vi "QD_Error_Logger.vi"(0 "State_and_Data_In":T1, 1 "Max_Queue_Size_In":i32=-1, 2 "Queue_Name_In":string, 5 "State_and_Data_N_In":T1[](array[typedef]), 7 "Time_Out_In_ms (-1)":i32, 11 "Error_In":errorcluster, 13 "Queue_Operation":T2=enum."Flush") -> (4 "State_and_Data_Out":T1, 15 "Error_Out":errorcluster)   [LabVIEW 2021]
doc: "Used to transfer data from one vi to another using queue."
uses:
  Controls/Queue_Operation_Select.ctl
  Controls/State_and_Data.ctl
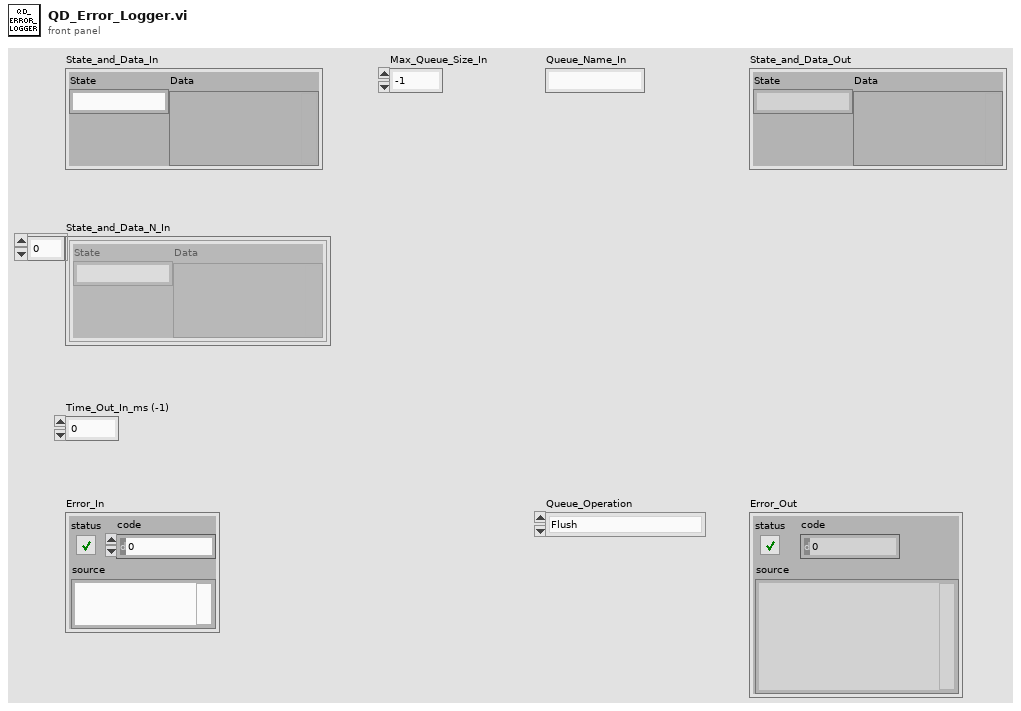
[diagram p1: front panel]
types:
  T1 = typedef "State_and_Data.ctl" = cluster{"State":string, "Data":variant}
  T2 = typedef "Queue_Operation_Select.ctl" = enum16{"Obtain_Queue", "Enqueue", "Enqueue_First", "Enqueue_N", "Lossy_Enqueue", "Preview", "Queue_Status", "Dequeue", "Flush", "Release_Queue"}
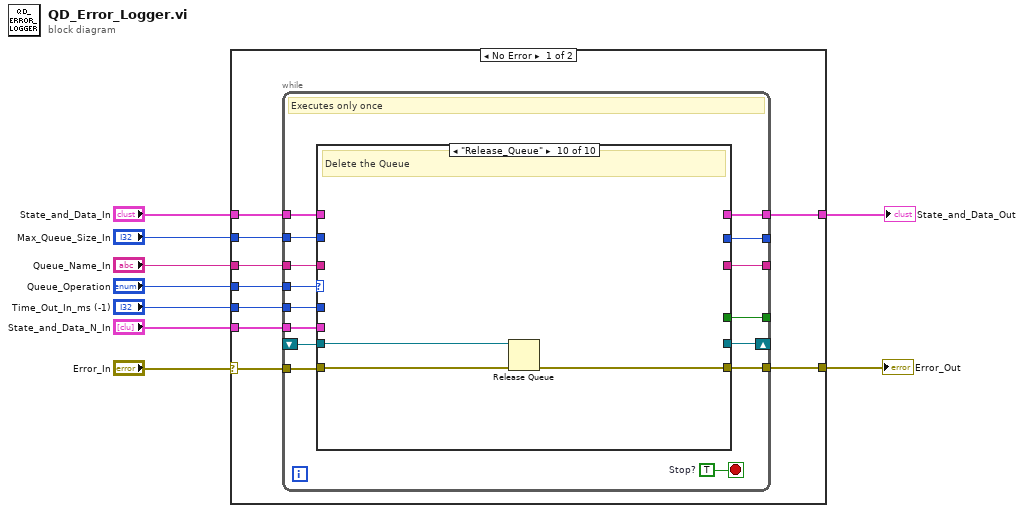
[diagram p0: block diagram]
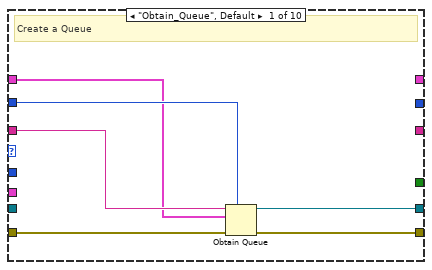
[diagram p2: hidden frame]
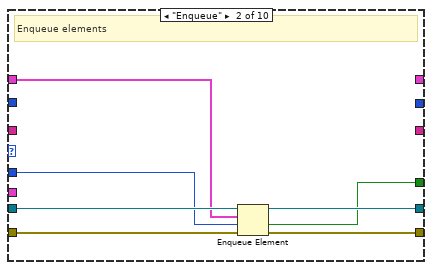
[diagram p3: hidden frame]
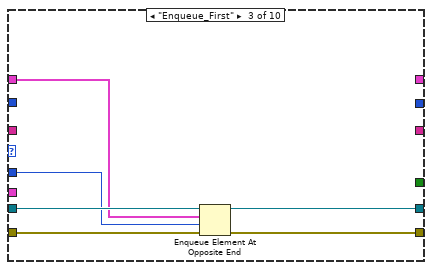
[diagram p4: hidden frame]
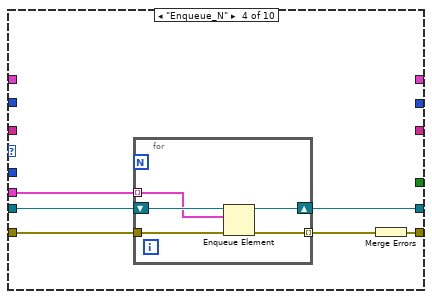
[diagram p5: hidden frame]
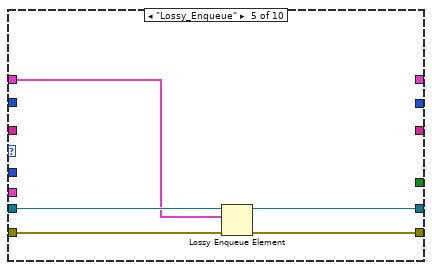
[diagram p6: hidden frame]
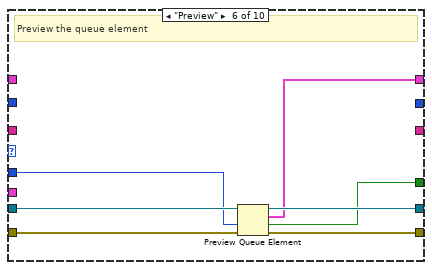
[diagram p7: hidden frame]
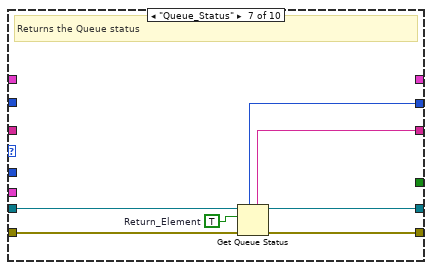
[diagram p8: hidden frame]
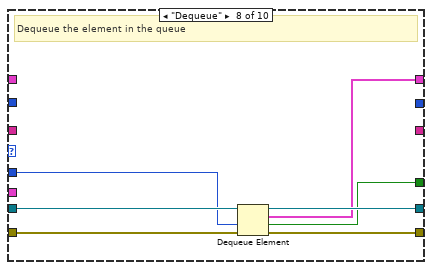
[diagram p9: hidden frame]
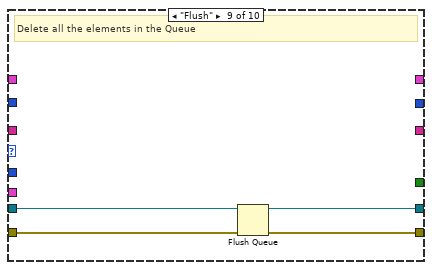
[diagram p10: hidden frame]
diagram:
  n1 = case shown="No Error" "Error_In" {
    selector: "Error_In" -> [w10 w97]
    tunnel: "Max_Queue_Size_In" -> [w18 _]
    tunnel: [w17 w97] -> w8
    tunnel: "Time_Out_In_ms (-1)" -> [w16 _]
    tunnel: "Queue_Operation" -> [w15 _]
    tunnel: "Queue_Name_In" -> [w14 _]
    tunnel: "State_and_Data_In" -> [w13 _]
    tunnel: [w12 _] -> w3
    tunnel: "State_and_Data_N_In" -> [w11 _]
    frame No Error {
      n2 = while {
        tunnel: w18 -> [w33]
        tunnel: w16 -> [w30]
        tunnel: [w28] -> _
        tunnel: w15 -> [w25]
        shift-right: [w26] -> _
        shift-left: _ -> [w22]
        tunnel: w13 -> [w31]
        tunnel: [w29] -> w12
        tunnel: w14 -> [w24]
        tunnel: [w27] -> _
        tunnel: w10 -> [w23]
        tunnel: [w32] -> w17
        tunnel: [w20] -> _
        tunnel: w11 -> [w19]
        stop <- w21 stop-if-true
        w21 = TRUE  # Stop?
        # "Executes only once"
        n3 = case shown="\"Release_Queue\"" w25 {
          tunnel: w23 -> [w39 w46 w52 w58 w67 w74 w81 w88 w92 w96]
          tunnel: w24 -> [w37 _ _ _ _ _ _ _ _ _]
          tunnel: w33 -> [w36 _ _ _ _ _ _ _ _ _]
          tunnel: [w34 w42 w47 w55 w66 w73 w80 w87 w91 _] -> w26
          tunnel: [w38 w45 w51 w53 w65 w72 w79 w85 w90 w95] -> w32
          tunnel: w22 -> [_ w44 w50 w56 w68 w75 w82 w89 w93 w94]
          tunnel: w31 -> [w35 w43 w49 _ w64 _ _ _ _ _]
          tunnel: w30 -> [_ w41 w48 _ _ w71 _ w84 _ _]
          tunnel: [_ _ _ _ _ w70 _ w86 _ _] -> w29
          tunnel: [_ _ _ _ _ _ w78 _ _ _] -> w28
          tunnel: [_ _ _ _ _ _ w77 _ _ _] -> w27
          tunnel: [_ w40 _ _ _ w69 _ w83 _ _] -> w20
          tunnel: w19 -> [_ _ _ w54 _ _ _ _ _ _]
          frame "Obtain_Queue", Default {
            # "Create a Queue"
            n4 = Obtain Queue(max queue size (-1, unlimited)=w36, name (unnamed)=w37, element data type=w35, error in (no error)=w39) -> (queue out=w34:refnum<queue>, error out=w38:errorcluster)  [unwired: 1 in, 1 out]
          }
          frame "Enqueue" {
            # "Enqueue elements"
            n5 = Enqueue Element(queue=w44, element=w43, timeout in ms (-1)=w41, error in (no error)=w46) -> (queue out=w42:refnum<queue>, timed out?=w40:bool, error out=w45:errorcluster)
          }
          frame "Enqueue_First" {
            n6 = Enqueue Element At Opposite End(queue=w50, element=w49, timeout in ms (-1)=w48, error in (no error)=w52) -> (queue out=w47:refnum<queue>, error out=w51:errorcluster)  [unwired: 1 out]
          }
          frame "Enqueue_N" {
            n7 = for {
              tunnel: w54 -> [w59] mode=indexing
              tunnel: w58 -> [w63]
              tunnel: [w62] -> w57 mode=indexing
              shift-right: [w60] -> w55
              shift-left: w56 -> [w61]
              n8 = Enqueue Element(queue=w61, element=w59, error in (no error)=w63) -> (queue out=w60:refnum<queue>, error out=w62:errorcluster)  [unwired: 1 in, 1 out]
            }
            n9 = Merge Errors(w57) -> (w53:errorcluster)
          }
          frame "Lossy_Enqueue" {
            n10 = Lossy Enqueue Element(queue=w68, element=w64, error in (no error)=w67) -> (queue out=w66:refnum<queue>, error out=w65:errorcluster)  [unwired: 2 out]
          }
          frame "Preview" {
            # "Preview the queue element"
            n11 = Preview Queue Element(queue=w75, timeout in ms (-1)=w71, error in (no error)=w74) -> (queue out=w73:refnum<queue>, element=w70:T1, timed out?=w69:bool, error out=w72:errorcluster)
          }
          frame "Queue_Status" {
            w76 = TRUE  # Return_Element
            # "Returns the Queue status"
            n12 = Get Queue Status(queue=w82, return elements? (F)=w76, error in (no error)=w81) -> (queue out=w80:refnum<queue>, queue name=w77:string, max queue size=w78:i32, error out=w79:errorcluster)  [unwired: 4 out]
          }
          frame "Dequeue" {
            # "Dequeue the element in the queue"
            n13 = Dequeue Element(queue=w89, timeout in ms (-1)=w84, error in (no error)=w88) -> (queue out=w87:refnum<queue>, element=w86:T1, timed out?=w83:bool, error out=w85:errorcluster)
          }
          frame "Flush" {
            # "Delete all the elements in the Queue"
            n14 = Flush Queue(queue=w93, error in (no error)=w92) -> (queue out=w91:refnum<queue>, error out=w90:errorcluster)  [unwired: 1 out]
          }
          frame "Release_Queue" {
            # "Delete the Queue"
            n15 = Release Queue(queue=w94, error in (no error)=w96) -> (error out=w95:errorcluster)  [unwired: 1 in, 2 out]
          }
        }
      }
    }
    frame Error {
    }
  }
  "Error_Out" <- w8
  "State_and_Data_Out" <- w3
